vi "CHKSUM计算 (子VI).vi"(11 "发送ASCII字符":string) -> (3 "CHECKSUM":u16 format="%xH")   [LabVIEW 2016, in "环境动力监测库.lvlib" / "空调库.lvlib"]
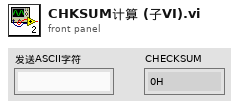
[diagram p1: front panel]
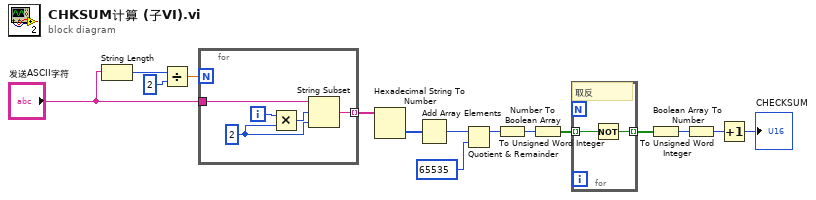
[diagram p0: block diagram]
diagram:
  n1 = String Length(string="发送ASCII字符") -> (length=w2:i32)
  n2 = Divide(x=w2, y=2) -> (x/y=w4:dbl)
  n3 = for {
    N: w4 -> [_]
    tunnel: "发送ASCII字符" -> [w20]
    tunnel: [w16] -> w5 mode=indexing
    i -> [w19]
    w18 = 2 ("长度（剩余）")
    n4 = Multiply(x=w19, y=w18) -> (x*y=w17:i32)
    n5 = String Subset(string=w20, offset (0)=w17, length (rest)=w18) -> (substring=w16:string)
  }
  n6 = Hexadecimal String To Number(string=w5) -> (number=w6:u32[])  [unwired: 2 in, 1 out]
  n7 = Add Array Elements(numeric array=w6) -> (sum=w13:u32)
  n8 = Quotient & Remainder(x=w13, y=u32 65535) -> (x-y*floor(x/y)=w11:u32)  [unwired: 1 out]
  n9 = To Unsigned Word Integer(number=w11) -> (unsigned 16bit integer=w10:u16)
  n10 = Number To Boolean Array(number=w10) -> (Boolean array=w15:bool[])
  n11 = for {
    tunnel: w15 -> [w22] mode=indexing
    tunnel: [w21] -> w9 mode=indexing
    # "取反"
    n12 = Not(x=w22) -> (.not. x?=w21:bool)
  }
  n13 = Boolean Array To Number(Boolean array=w9) -> (number=w8:u32)
  n14 = To Unsigned Word Integer(number=w8) -> (unsigned 16bit integer=w7:u16)
  n15 = Increment(x=w7) -> (x+1=→"CHECKSUM":u16)
